vi "Read Test Data (Program Mode).vi"(0 "VISA resource name":refnum<visa-resource-name>, 11 "error in (no error)":errorcluster) -> (4 "VISA resource name out":refnum<visa-resource-name>, 6 "Test Meter Data Output":T1 {"Frequency (Hz)" format="%.1f"; "Voltage (V)" format="%.1f"; "RMS Current (A)" format="%.3f"; "Power (W)" format="%.1f"; "Peak Current (A)" format="%.1f"; "Power Factor" format="%.3f"; "Timer (s)" format="%.1f"}, 15 "error out":errorcluster)   [LabVIEW 2014, in "eec 6700.lvlib"]
doc: "Reads the Program mode <B>active data being displayed on the LCD display</B> while the test is in process. It also gives the last data taken when the test sequence completed. \n\nIn Program Mode the output data cluster has the following data.\n\n1. Memory\n2. Step\n3. Timer (s)\n4. Frequency (Hz)\n5. Voltage (V)\n6. RMS Current (A)\n7. Peak Current (A)\n8. Power (W)\n9. Power Factor\n10. Status"
uses:
  <instrlib>/eec 6700/eec 6700.lvlib
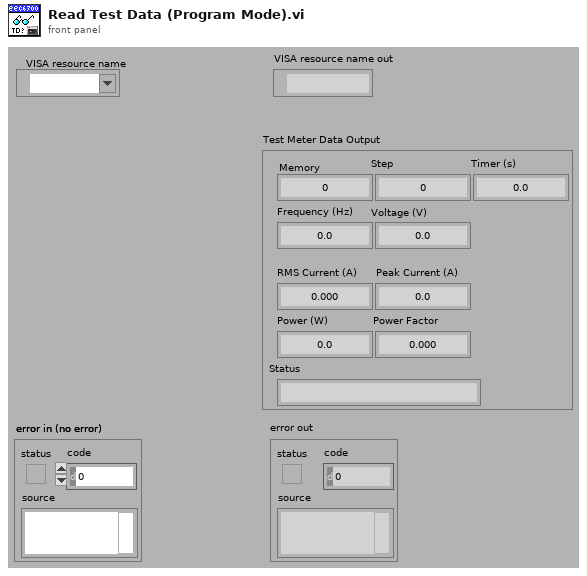
[diagram p1: front panel]
types:
  T1 = cluster{"Memory":dbl, "Step":dbl, "Timer (s)":dbl, "Frequency (Hz)":dbl, "Voltage (V)":dbl, "RMS Current (A)":dbl, "Peak Current (A)":dbl, "Power (W)":dbl, "Power Factor":dbl, "Status":string}
  T2 = cluster{"Memory":i32, "Step":i32, "Timer":dbl, "Frequency":dbl, "Volt":dbl, "Current":dbl, "Peak Current":dbl, "Power":dbl, "Power Factor":dbl, "Status":string}
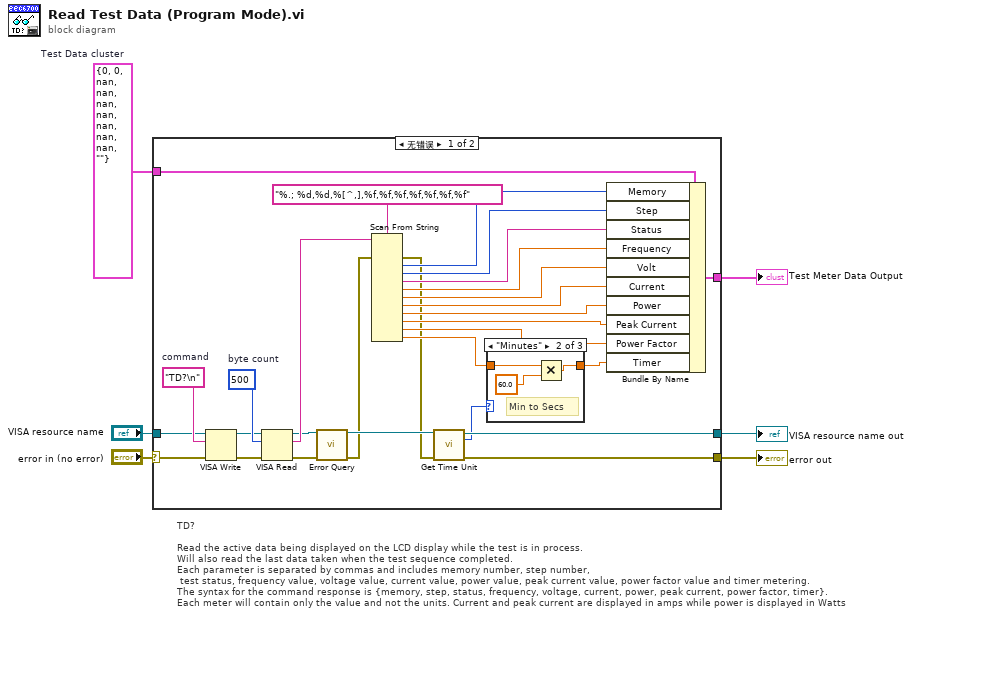
[diagram p0: block diagram]
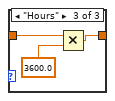
[diagram p3: hidden frame]
diagram:
  w2 = T2 {"Memory"=0, "Step"=0, "Timer"=nan, "Frequency"=nan, "Volt"=nan, "Current"=nan, "Peak Current"=nan, "Power"=nan, "Power Factor"=nan, "Status"=""}  # Test Data cluster
  # "TD?\n\nRead the active data being displayed on the LCD display while the test is in process. \nWill also read the last data taken when the test sequence completed. \nEach parameter is separated by commas and includes memory number, step number,\n test status, frequency value, voltage value, current value, power value, peak current value, power factor value and timer metering. \nThe syntax for the command response is {memory, step, status, frequency, voltage, current, power, peak current, power factor, timer}. \nEach meter will contain only the value and not the units. Current and peak current are displayed in amps while power is displayed in Watts"
  n1 = case shown="无错误" "error in (no error)" {
    selector: "error in (no error)" -> [w7 w44]
    tunnel: "VISA resource name" -> [w8 w45]
    tunnel: [w30 w45] -> w4
    tunnel: [w31 w44] -> w3
    tunnel: [w34 w43] -> w1
    tunnel: w2 -> [w33 w43]
    frame No Error {
      w32 = "TD?\n"  # command
      w35 = u32 500  # byte count
      n2 = VISA Write(VISA resource name=w8, write buffer=w32, error in (no error)=w7) -> (VISA resource name out=w11:refnum<visa-resource-name>, error out=w10:errorcluster)  [unwired: 1 out]
      n3 = VISA Read(VISA resource name=w11, byte count=w35, error in (no error)=w10) -> (VISA resource name out=w16:refnum<visa-resource-name>, read buffer=w17:string, error out=w12:errorcluster)  [unwired: 1 out]
      n4 = call <instrlib>:"Error Query.vi"("VISA resource name"=w16, "error in (no error)"=w12) -> ("VISA resource name out"=w15:refnum<visa-resource-name>, "error out"=w14:errorcluster)  [unwired: 10 in, 2 out]
      n5 = Scan From String(format string="%.; %d,%d,%[^,],%f,%f,%f,%f,%f,%f,%f", input string=w17, error in=w14) -> (error out=w13:errorcluster, output 1=w27:i32, output 2=w26:i32, output 3=w25:string, output 4=w24:dbl, output 5=w23:dbl, output 6=w22:dbl, output 7=w21:dbl, output 8=w20:dbl, output 9=w19:dbl, output 10=w18:dbl)  [unwired: 11 in, 2 out]
      n6 = call <instrlib>:"Get Time Unit.vi"("VISA resource name"=w15, "error in (no error)"=w13) -> ("VISA resource name out"=w30:refnum<visa-resource-name>, "Time Unit"=w9:enum16{"Seconds", "Minutes", "Hours"}, "error out"=w31:errorcluster)  [unwired: 11 in]
      n7 = case shown="\"Minutes\"" w9 {
        tunnel: [w36 w38 w41] -> w29
        tunnel: w18 -> [w36 w37 w40]
        frame "Seconds" {
        }
        frame "Minutes" {
          # "Min to Secs"
          n8 = Multiply(x=w37, y=60.0) -> (x*y=w38:dbl)
        }
        frame "Hours" {
          n9 = Multiply(x=w40, y=3600.0) -> (x*y=w41:dbl)
        }
      }
      n10 = Bundle By Name(cluster=w33, "Memory"=w27, "Step"=w26, "Status"=w25, "Frequency"=w24, "Volt"=w23, "Current"=w22, "Power"=w21, "Peak Current"=w20, "Power Factor"=w19, "Timer"=w29) -> (w34:T2)
    }
    frame Error {
    }
  }
  "VISA resource name out" <- w4
  "error out" <- w3
  "Test Meter Data Output" <- w1
